vi "WriteResultLine.vi"(8 "error in (no error)":errorcluster, 11 "AnalysisPluginsBase in":refnum<class "AnalysisPluginsBase.lvclass">) -> (0 "error out":errorcluster, 3 "AnalysisPluginsBase out":refnum<class "AnalysisPluginsBase.lvclass">)   [LabVIEW 2014, in "AnalysisPlugins.lvlib" / "AnalysisPluginsBase.lvclass"]
uses:
  AnalysisPluginsBase.lvclass
  AnalysisPluginsBase.lvclass/AnalysisPluginsBase.ctl
  Accessors/Read FileName.vi
  Accessors/Read Result.vi
  <vilib>/Utility/file.llb/Write To Spreadsheet File (DBL).vi
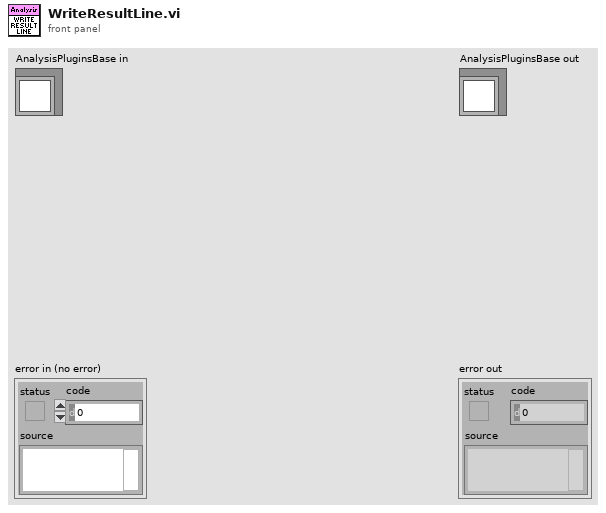
[diagram p1: front panel]
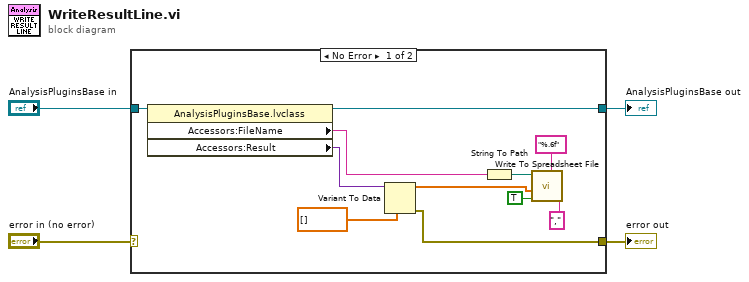
[diagram p0: block diagram]
diagram:
  n1 = case shown="No Error" "error in (no error)" {
    selector: "error in (no error)" -> [_ w17]
    tunnel: [w5 w17] -> w3
    tunnel: [w14 w16] -> w1
    tunnel: "AnalysisPluginsBase in" -> [w15 w16]
    frame No Error {
      n2 = property class="AnalysisPluginsBase.lvclass"(reference=w15) -> (reference out=w14:refnum<class "AnalysisPluginsBase.lvclass">, "Accessors:FileName"=w12:string, "Accessors:Result"=w8:variant)  [unwired: 1 in, 1 out]
      n3 = Variant To Data(type=dbl[] [], Variant=w8) -> (data=w6:dbl[], error out=w5:errorcluster)  [unwired: 1 in]
      n4 = String To Path(string=w12) -> (path=w11:path)
      n5 = call-poly <vilib>:"Write To Spreadsheet File.vi"("delimiter (\\t)"="," ("delimiter (\\t)"), "format (%.3f)"="%.6f", "append to file? (new file:F)"=TRUE, "1D data"=w6, "file path (dialog if empty)"=w11) -> ()  [unwired: 3 in, 1 out]
    }
    frame Error {
    }
  }
  "error out" <- w3
  "AnalysisPluginsBase out" <- w1
